vi "CANOpen Import SDO.vi"(8 "error in (no error)":errorcluster, 10 "Display format":T2, 11 "SDO Parameters in":T1[](array[typedef]) {"Sub-Index (0)" format="%.0x"; "Object Index" format="%.0x"; "Block Data" format="%.0x"}) -> (0 "error out":errorcluster, 3 "SDO Parameters":T1[](array[typedef]) {"Sub-Index (0)" format="%.0x"; "Object Index" format="%.0x"; "Block Data" format="%.0x"})   [LabVIEW 2021, in "CANOpen Addon System Explorer.lvlib"]
uses:
  CANOpen Addon System Explorer.lvlib
  CANOpen_SDO data format.ctl
  Shared/CANOpen_SDO Settings.ctl
  Shared/CANOpen Addon Shared.lvlib
panel:
  out "spreadsheet string":string
  # "LSB"
  # "MSB"
  # "LSB"
  # "MSB"
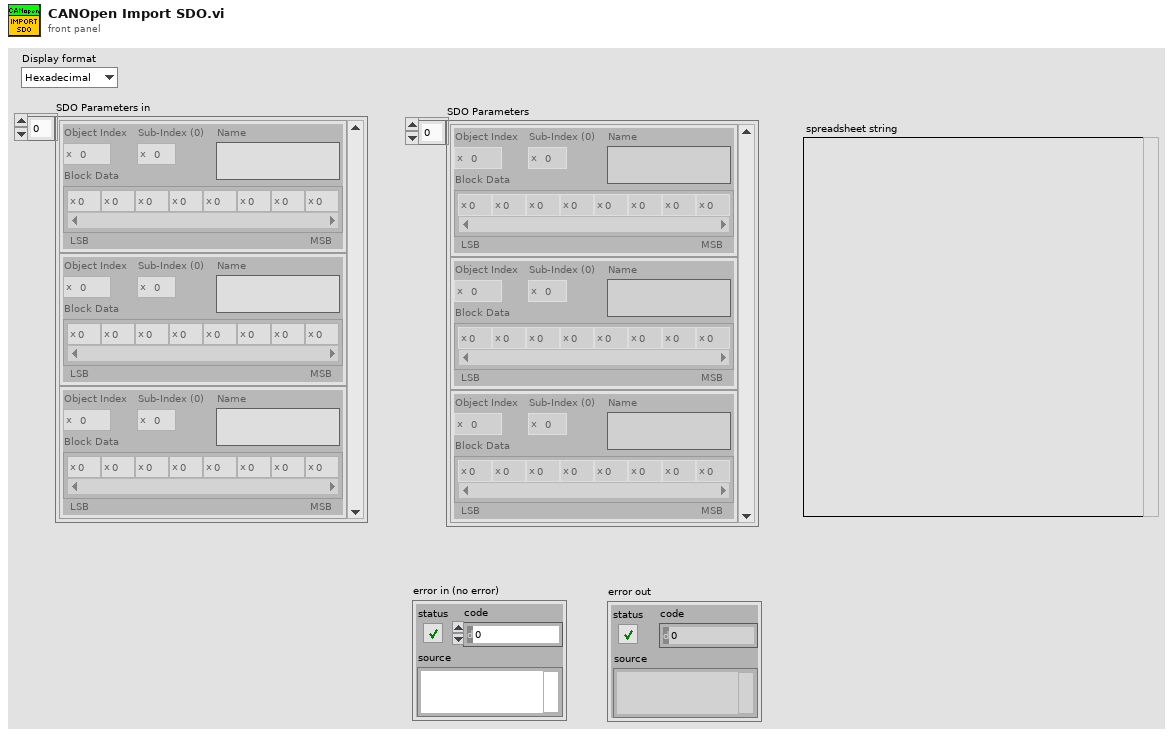
[diagram p1: front panel]
types:
  T1 = typedef "CANOpen Addon Shared.lvlib/CANOpen_SDO Settings.ctl" = cluster{"Object Index":u16, "Sub-Index (0)":u8, "Block Data":u8[], "Name":string}
  T2 = typedef "CANOpen Addon System Explorer.lvlib/CANOpen_SDO data format.ctl" = enum16{"Hexadecimal", "Decimal"}
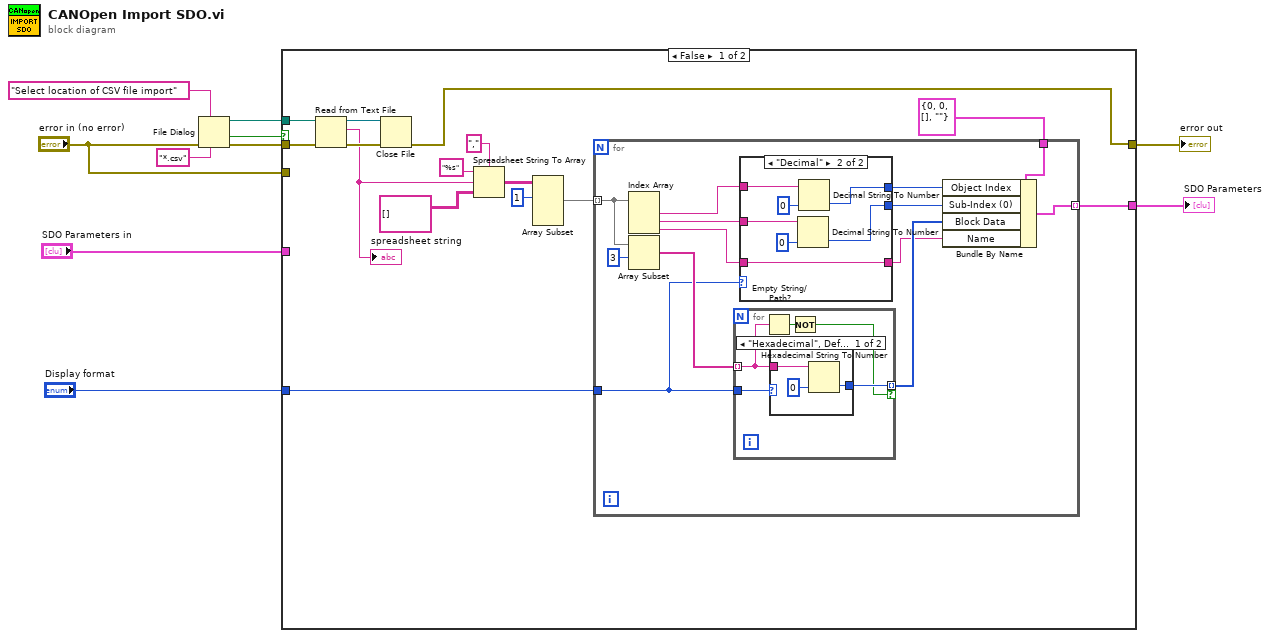
[diagram p0: block diagram]
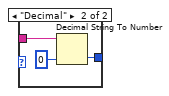
[diagram p2: hidden frame]
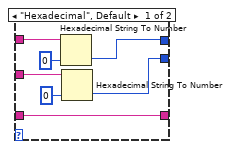
[diagram p3: hidden frame]
diagram:
  n1 = File Dialog(6:"*.csv" ("pattern (all files)"), 7:"Select location of CSV file import" ("prompt"), 8:"error in (no error)") -> (0:w7:errorcluster, 1:w8:bool, 3:w4:path)  [unwired: 4 in, 1 out]
  n2 = case shown="False" w8 {
    tunnel: w7 -> [w23 _]
    tunnel: [w11 w65] -> w6
    tunnel: "error in (no error)" -> [_ w65]
    tunnel: w4 -> [w24 _]
    tunnel: "SDO Parameters in" -> [_ w64]
    tunnel: [w16 w64] -> w2
    tunnel: "Display format" -> [w25 _]
    frame False {
      n3 = Read from Text File(file (use dialog)=w24, error in=w23) -> (refnum out=w21:refnum<file>, text=w17:string, error out=w22:errorcluster)  [unwired: 2 in, 1 out]
      "spreadsheet string" <- w17
      n4 = Close File(refnum=w21, error in=w22) -> (error out=w11:errorcluster)  [unwired: 1 out]
      n5 = Spreadsheet String To Array(delimiter (Tab)=",", format string="%s", spreadsheet string=w17, array type (2D Dbl)=string[][] [] ("appended array")) -> (array=w14:string[][])
      n6 = Array Subset(array=w14, index (row)=1 ("index")) -> (w13:string[][])  [unwired: 3 in]
      n7 = for {
        tunnel: w25 -> [w28]
        tunnel: T1 {"Object Index"=0, "Sub-Index (0)"=0, "Block Data"=[], "Name"=""} -> [w38]
        tunnel: [w37] -> w16 mode=indexing
        tunnel: w13 -> [w36] mode=indexing
        n8 = Index Array(array=w36) -> (element #1=w33:string, element #2=w30:string, element #3=w26:string)  [unwired: 3 in]
        n9 = Array Subset(array=w36, index=3) -> (w34:string[])  [unwired: 1 in]
        n10 = for {
          tunnel: w34 -> [w41] mode=indexing
          tunnel: [w43] -> w29 mode=indexing if=w39
          tunnel: w28 -> [w42]
          n11 = Empty String/Path?(string/path=w41) -> (empty?=w40:bool)
          n12 = case shown="\"Hexadecimal\", Default" w42 {
            tunnel: [w45 w48] -> w43
            tunnel: w41 -> [w44 w47]
            frame "Hexadecimal", Default {
              n13 = Hexadecimal String To Number(string=w44, default (0uL)=u8 0 ("default (0 U32)")) -> (number=w45:u8)  [unwired: 1 in, 1 out]
            }
            frame "Decimal" {
              n14 = Decimal String To Number(string=w47, default (0L)=u8 0 ("default (0 I32)")) -> (number=w48:u8)  [unwired: 1 in, 1 out]
            }
          }
          n15 = Not(x=w40) -> (.not. x?=w39:bool)
        }
        n16 = case shown="\"Decimal\"" w28 {
          tunnel: [w54 w60] -> w31
          tunnel: w33 -> [w55 w63]
          tunnel: [w56 w62] -> w32
          tunnel: w30 -> [w53 w61]
          tunnel: [w50 w57] -> w27
          tunnel: w26 -> [w50 w57]
          frame "Hexadecimal", Default {
            n17 = Hexadecimal String To Number(string=w55, default (0uL)=u16 0 ("default (0 U32)")) -> (number=w56:u16)  [unwired: 1 in, 1 out]
            n18 = Hexadecimal String To Number(string=w53, default (0uL)=u8 0 ("default (0 U32)")) -> (number=w54:u8)  [unwired: 1 in, 1 out]
          }
          frame "Decimal" {
            n19 = Decimal String To Number(string=w61, default (0L)=u8 0 ("default (0 I32)")) -> (number=w60:u8)  [unwired: 1 in, 1 out]
            n20 = Decimal String To Number(string=w63, default (0L)=u16 0 ("default (0 I32)")) -> (number=w62:u16)  [unwired: 1 in, 1 out]
          }
        }
        n21 = Bundle By Name(cluster=w38, "Object Index"=w32, "Sub-Index (0)"=w31, "Block Data"=w29, "Name"=w27) -> (w37:T1)
      }
    }
    frame True {
    }
  }
  "SDO Parameters" <- w2
  "error out" <- w6
